vi "rsscope_FormatUSBPDPacketTypeString_WriteCallback.vi"(5 "Attribute":T1={"Identifier"="", "Descriptive Name"="", "Data Type"=enum."Integer 32", "Command"="", "Access"=enum."Read/Write", "Range Table"="", "Read Callback"="", "Write Callback"="", "Supported Models"="", "Instrument Options"="", "Index"=0, "OPC Wait"=FALSE, "No Status Check"=FALSE, "Cache Only"=FALSE}, 7 "Repeated Capability":string, 8 "error in (no error)":errorcluster, 10 "Attribute Value String":string, 11 "VISA resource name":refnum<visa-resource-name>) -> (0 "error out":errorcluster, 3 "VISA resource name out":refnum<visa-resource-name>)   [LabVIEW 2018]
doc: "This VI sets the attribute value.\n\nThis is a low-level VI that you can use to set the values of instrument-specific properties and inherent IVI properties. If the property represents an instrument state, this VI performs instrument I/O in the following cases:\n\n- State caching is disabled for the entire session or for the particular property.\n\n- State caching is enabled and the currently cached value is invalid or is different than the value you specify. \n\nThis instrument driver contains high-level VIs that set most of the instrument properties. It is best to use the high-level driver VIs as much as possible. They handle order dependencies and multithread locking for you. In addition, they perform status checking only after setting all of the properties. In contrast, when you set multiple properties using the SetAttribute VIs, the VIs check the instrument status after each call.\n\nAlso, when state caching is enabled, the high-level VIs that configure multiple properties perform instrument I/O only for the properties whose value you change. Thus, you can safely call the high-level VIs without the penalty of redundant instrument I/O."
uses:
  rsidr_core.llb/type_Attribute.ctl
  rsidr_core.llb/type_Attribute_Data_Type.ctl
  rsidr_core.llb/type_ReadWriteAccess.ctl
  rsidr_core.llb/rsscope_rsidr_core.lvlib
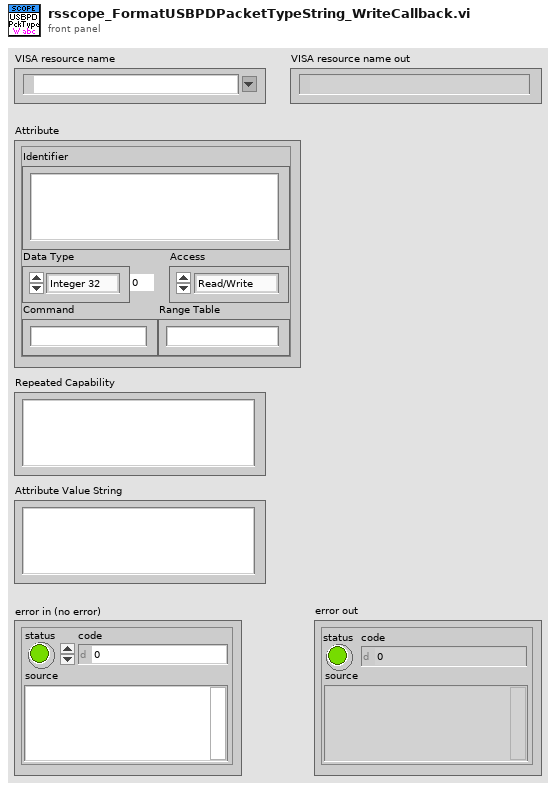
[diagram p1: front panel]
types:
  T1 = typedef "rsscope_rsidr_core.lvlib/type_Attribute.ctl" = cluster{"Identifier":string, "Descriptive Name":string, "Data Type":T2, "Command":string, "Access":T3, "Range Table":string, "Read Callback":string, "Write Callback":string, "Supported Models":string, "Instrument Options":string, "Index":i32, "OPC Wait":bool, "No Status Check":bool, "Cache Only":bool}
  T2 = typedef "rsscope_rsidr_core.lvlib/type_Attribute_Data_Type.ctl" = enum16{"Integer 32", "Double", "String", "Boolean", "None", "Integer 64", "RawString"}
  T3 = typedef "rsscope_rsidr_core.lvlib/type_ReadWriteAccess.ctl" = enum16{"Read Only", "Write Only", "Read/Write"}
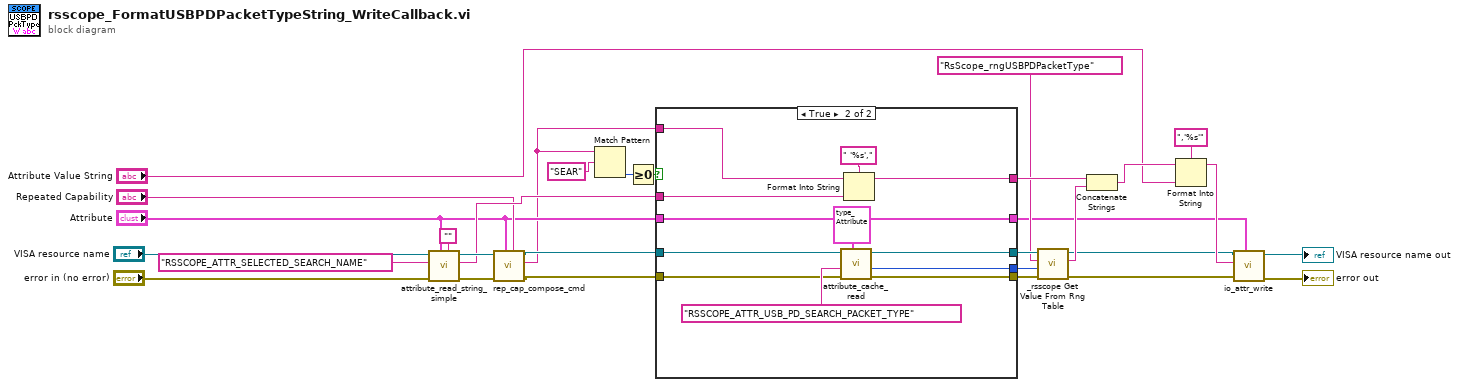
[diagram p0: block diagram]
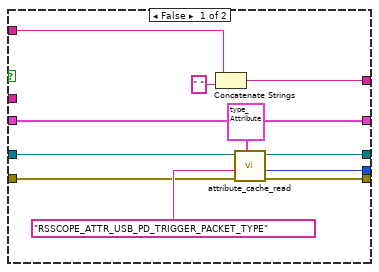
[diagram p2: hidden frame]
diagram:
  n1 = call "attribute_read_string_simple.vi"("Repeated Capability"="" ("Empty String Constant"), "Attribute"="Attribute", "error in"="error in (no error)", "Direct Attribute ID (\"\")"="RSSCOPE_ATTR_SELECTED_SEARCH_NAME" ("Direct Attribute ID (\"\")"), "VISA resource name"="VISA resource name") -> ("error out"=w24:errorcluster, "String out"=w8:string, "VISA resource name out"=w23:refnum<visa-resource-name>)  [unwired: 4 in]
  n2 = call "rep_cap_compose_cmd.vi"("Repeated Capability"="Repeated Capability", "Attribute"="Attribute", "error in"=w24, "VISA resource name"=w23) -> ("error out"=w12:errorcluster, "Command out"=w1:string, "VISA resource name out"=w11:refnum<visa-resource-name>)  [unwired: 5 in]
  n3 = Match Pattern(string=w1, regular expression="SEAR" ("true string")) -> (offset past match=w15:i32)  [unwired: 1 in, 3 out]
  n4 = Greater Or Equal To 0?(x=w15) -> (x >= 0?=w14:bool)
  n5 = case shown="True" w14 {
    tunnel: w8 -> [_ w52]
    tunnel: [w41 w51] -> w21
    tunnel: w1 -> [w31 w42]
    tunnel: w11 -> [w35 w46]
    tunnel: w12 -> [w36 w47]
    tunnel: [w32 w44] -> w20
    tunnel: [w33 w45] -> w19
    tunnel: [w34 w43] -> w18
    tunnel: "Attribute" -> [w39 w50]
    tunnel: [w39 w50] -> w5
    frame False {
      n6 = Concatenate Strings(w31, " " ("string")) -> (w41:string)
      n7 = call "attribute_cache_read.vi"("Attribute"=T1 {"Identifier"="", "Descriptive Name"="", "Data Type"=enum."Integer 32", "Command"="", "Access"=enum."Read/Write", "Range Table"="", "Read Callback"="", "Write Callback"="", "Supported Models"="", "Instrument Options"="", "Index"=0, "OPC Wait"=FALSE, "No Status Check"=FALSE, "Cache Only"=FALSE}, "error in"=w36, "Direct Attribute ID (Attribute cluster)"="RSSCOPE_ATTR_USB_PD_TRIGGER_PACKET_TYPE" ("Direct Attribute ID (\"\")"), "VISA resource name"=w35) -> ("error out"=w33:errorcluster, "Int32 out"=w34:i32, "VISA resource name out"=w32:refnum<visa-resource-name>)  [unwired: 5 out]
    }
    frame True {
      n8 = call "attribute_cache_read.vi"("Attribute"=T1 {"Identifier"="", "Descriptive Name"="", "Data Type"=enum."Integer 32", "Command"="", "Access"=enum."Read/Write", "Range Table"="", "Read Callback"="", "Write Callback"="", "Supported Models"="", "Instrument Options"="", "Index"=0, "OPC Wait"=FALSE, "No Status Check"=FALSE, "Cache Only"=FALSE}, "error in"=w47, "Direct Attribute ID (Attribute cluster)"="RSSCOPE_ATTR_USB_PD_SEARCH_PACKET_TYPE" ("Direct Attribute ID (\"\")"), "VISA resource name"=w46) -> ("error out"=w45:errorcluster, "Int32 out"=w43:i32, "VISA resource name out"=w44:refnum<visa-resource-name>)  [unwired: 5 out]
      n9 = Format Into String(format string=" '%s',", initial string=w42, w52) -> (resulting string=w51:string)  [unwired: 1 in, 1 out]
    }
  }
  n10 = call "_rsscope Get Value From Rng Table.vi"("error in (no error)"=w19, "Value"=w18, "Range Table Name"="RsScope_rngUSBPDPacketType", "VISA resource name"=w20) -> ("error out"=w10:errorcluster, "Output Enum value"=w16:string, "VISA resource name out"=w9:refnum<visa-resource-name>)  [unwired: 5 in]
  n11 = Concatenate Strings(w21, w16) -> (w4:string)
  n12 = Format Into String(format string=",'%s'", initial string=w4, "Attribute Value String") -> (resulting string=w22:string)  [unwired: 1 in, 1 out]
  n13 = call "io_attr_write.vi"("Attribute"=w5, "error in"=w10, "write buffer"=w22, "VISA resource name"=w9) -> ("error out"=→"error out":errorcluster, "VISA resource name out"=→"VISA resource name out":refnum<visa-resource-name>)  [unwired: 6 in]
